vi "Save Screen Shot.vi"(5 "Enable Ink Saver (F: Disable)":bool, 6 "Color Palette (0: Color)":u16(ring) items=["Color", "Grayscale"], 7 "Include Factors (F: Disable)":bool, 8 "error in (no error)":errorcluster, 9 "Format (0: 24-bit Bitmap)":u16(ring) items=["24-bit Bitmap", "8-bit Bitmap", "24-bit PNG", "Bitmap"], 10 "File Name (Empty String)":string, 11 "VISA resource name":refnum<visa-resource-name>) -> (0 "error out":errorcluster, 3 "VISA resource name out":refnum<visa-resource-name>)   [LabVIEW 2015, in "Agilent 2000 3000 X-Series.lvlib"]
doc: "Saves a screen shot of the scope display to a file."
uses:
  Agilent 2000 3000 X-Series.lvlib
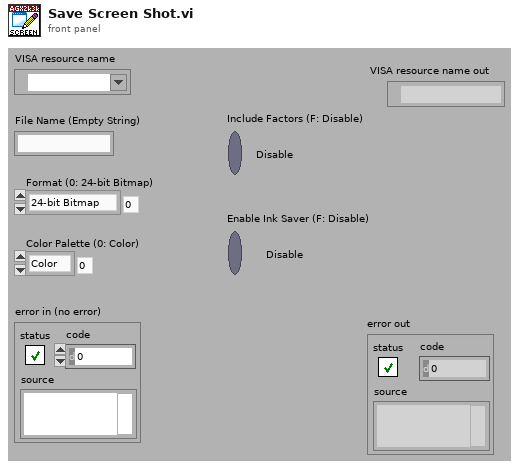
[diagram p1: front panel]
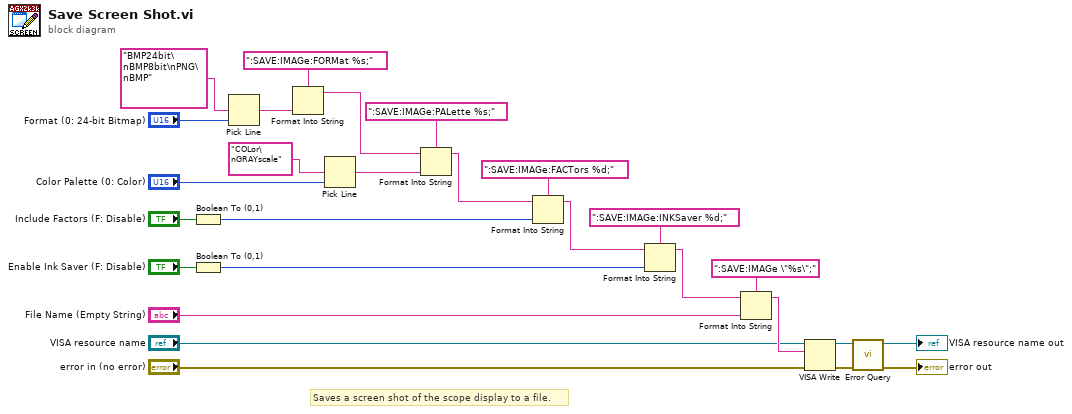
[diagram p0: block diagram]
diagram:
  # "Saves a screen shot of the scope display to a file."
  n1 = Boolean To (0,1)(Boolean="Include Factors (F: Disable)") -> (0, 1=w13:i16)
  n2 = Boolean To (0,1)(Boolean="Enable Ink Saver (F: Disable)") -> (0, 1=w18:i16)
  n3 = Pick Line(multi-line string="BMP24bit\nBMP8bit\nPNG\nBMP", line index="Format (0: 24-bit Bitmap)") -> (output string=w6:string)  [unwired: 1 in]
  n4 = Format Into String(format string=":SAVE:IMAGe:FORMat %s;", w6) -> (resulting string=w7:string)  [unwired: 2 in, 1 out]
  n5 = Pick Line(multi-line string="COLor\nGRAYscale", line index="Color Palette (0: Color)") -> (output string=w10:string)  [unwired: 1 in]
  n6 = Format Into String(format string=":SAVE:IMAGe:PALette %s;", initial string=w7, w10) -> (resulting string=w12:string)  [unwired: 1 in, 1 out]
  n7 = Format Into String(format string=":SAVE:IMAGe:FACTors %d;", initial string=w12, w13) -> (resulting string=w14:string)  [unwired: 1 in, 1 out]
  n8 = Format Into String(format string=":SAVE:IMAGe:INKSaver %d;", initial string=w14, w18) -> (resulting string=w20:string)  [unwired: 1 in, 1 out]
  n9 = Format Into String(format string=":SAVE:IMAGe \"%s\";", initial string=w20, "File Name (Empty String)") -> (resulting string=w23:string)  [unwired: 1 in, 1 out]
  n10 = VISA Write(VISA resource name="VISA resource name", write buffer=w23, error in (no error)="error in (no error)") -> (VISA resource name out=w24:refnum<visa-resource-name>, error out=w25:errorcluster)  [unwired: 1 out]
  n11 = call "Error Query.vi"("error in (no error)"=w25, "VISA resource name"=w24) -> ("error out"=→"error out":errorcluster, "VISA resource name out"=→"VISA resource name out":refnum<visa-resource-name>)  [unwired: 6 in, 2 out]
